vi "Unit test - BackUp on DB Size Multiples.vi"(8 "error in (no error)":errorcluster, 9 "Actual DB size":i32, 10 "Max DB Size":i32, 11 "Data Size":i32) -> (0 "error out":errorcluster, 3 "Limits":i32[](array[numeric]))   [LabVIEW 2014]
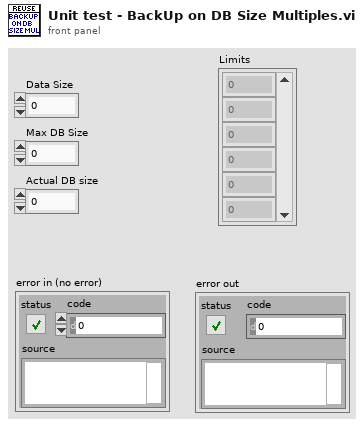
[diagram p1: front panel]
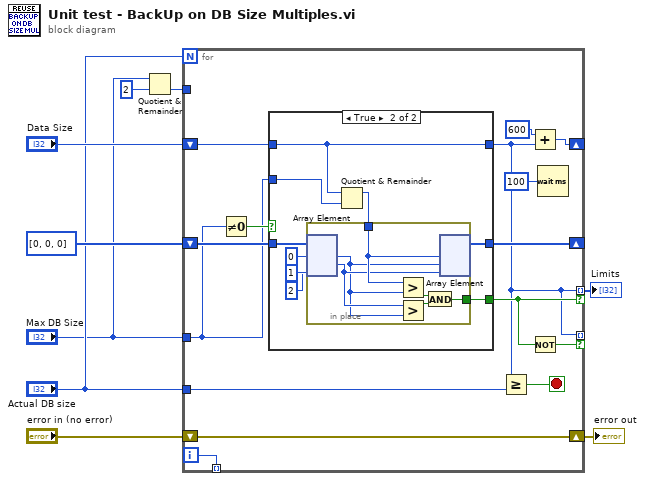
[diagram p0: block diagram]
diagram:
  n1 = Quotient & Remainder(x="Max DB Size", y=2) -> (floor(x/y)=w3:i32)  [unwired: 1 out]
  n2 = for {
    N: "Actual DB size" -> [_]
    tunnel: "Max DB Size" -> [w15]
    shift-right: [w24] -> _
    shift-left: "Data Size" -> [w23]
    tunnel: [w12] -> w8 mode=indexing if=w14
    shift-right: [w20] -> _
    shift-left: i32[] [0, 0, 0] ("Backup Size Circular Buf") -> [w21]
    tunnel: "Actual DB size" -> [w18]
    tunnel: [w16] -> _ mode=indexing
    tunnel: [w12] -> _ mode=indexing if=w13
    tunnel: w3 -> [_]
    shift-right: [w11] -> w1
    shift-left: "error in (no error)" -> [w11]
    i -> [w16]
    stop <- w17 stop-if-true
    n3 = Not Equal To 0?(x=w15) -> (x != 0?=w22:bool)
    n4 = case shown="True" w22 {
      tunnel: w15 -> [_ w35]
      tunnel: w21 -> [w26 w34]
      tunnel: [w26 w32] -> w20
      tunnel: w23 -> [w25 w27]
      tunnel: [_ w28] -> w14
      tunnel: [w25 w27] -> w12
      frame False {
      }
      frame True {
        n5 = Quotient & Remainder(x=w27, y=w35) -> (x-y*floor(x/y)=w33:i32)  [unwired: 1 out]
        n6 = in-place {
          in-place-border: w33 -> [w41]
          in-place-border: [w36] -> w28
          n7 = in-place-array #1(w34, 0, 1, 2) -> (w39:i32, w40:i32)  [unwired: 1 out]
          n8 = Greater?(x=w41, y=w39) -> (0:w37:bool)
          n9 = Greater?(x=w40, y=w39) -> (0:w38:bool)
          n10 = And(x=w37, y=w38) -> (x .and. y?=w36:bool)
          n11 = in-place-array #1(w41, w39, w40) -> (w32:i32[])  [unwired: 3 out]
        }
      }
    }
    n12 = Greater Or Equal?(x=w12, y=w18) -> (x >= y?=w17:bool)
    n13 = Add(x=600, y=w12) -> (x+y=w24:i32)
    n14 = Not(x=w14) -> (.not. x?=w13:bool)
    n15 = Wait (ms)(milliseconds to wait=u32 100) -> ()  [unwired: 1 out]
  }
  "Limits" <- w8
  "error out" <- w1
